vi "Construct PDU.vi"(8 "error in (no error)":errorcluster, 10 "data":u8[](array[numeric]), 11 "function":u8(ring) items=["Read Discrete Inputs"=2, "Read Coils"=1, "Write Single Coil"=5, "Write Multiple Coils"=15, "Read Input Register"=4, "Read Holding Registers"=3, "Write Single Register"=6, "Write Multiple Registers"=16, "Read/Write Multiple Registers"=23, "Mask Write Register"=22, "Read FIFO Queue"=24, "Read File Record"=20, "Write File Record"=21, "Read Exception Status"=7, "Diagnostic"=8, "Get Com Event Counter"=11, "Get Com Event Log"=12, "Report Slave ID"=17, "Read Device Identification"=43]) -> (0 "error out":errorcluster, 3 "Modbus data unit out":refnum<class "Modbus Data Unit (PDU).lvclass">)   [LabVIEW 2020, in "SubVIs.lvlib" / "Modbus Data Unit (PDU).lvclass"]
uses:
  <vilib>/Modbus/subvis/Modbus Data Unit (PDU)/Modbus Data Unit (PDU).lvclass
  <vilib>/Modbus/subvis/Modbus Data Unit (PDU)/Modbus Data Unit (PDU).lvclass/Modbus Data Unit (PDU).ctl
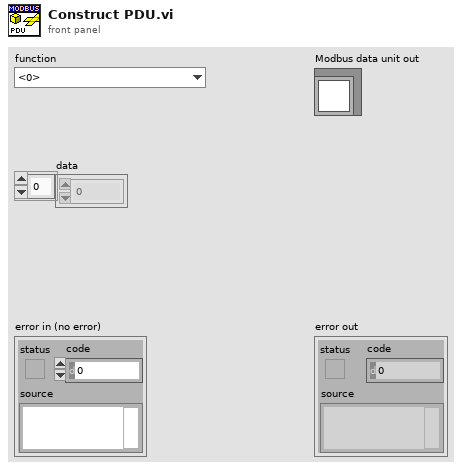
[diagram p1: front panel]
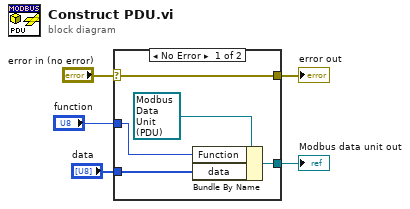
[diagram p0: block diagram]
diagram:
  n1 = case shown="No Error" "error in (no error)" {
    selector: "error in (no error)" -> [w6 w11]
    tunnel: [w10 _] -> w5
    tunnel: "function" -> [w9 _]
    tunnel: "data" -> [w8 _]
    tunnel: [w6 w11] -> w1
    frame No Error {
      n2 = Bundle By Name(cluster=refnum<class "Modbus Data Unit (PDU).lvclass"> refnum ("modbus data unit"), "Function"=w9, "data"=w8) -> (w10:refnum<class "Modbus Data Unit (PDU).lvclass">)
    }
    frame Error {
    }
  }
  "error out" <- w1
  "Modbus data unit out" <- w5
